vi "GetDiscoveredDevices.vi"(0 "CmdLib In":refnum<k24>, 7 "Master Count":i32, 9 "DeviceKey List":string[](array[string]), 11 "error in":errorcluster) -> (4 "CmdLib Out":refnum<k24>, 6 "Device Array":T1(array[cluster]), 15 "error out":errorcluster)   [LabVIEW 2013]
uses:
  C:/GEECS/Developers Version/source/Device Driver/Picomotor8742dotNet/NewFocus/CmdLib.dll
  CmdLib.dll
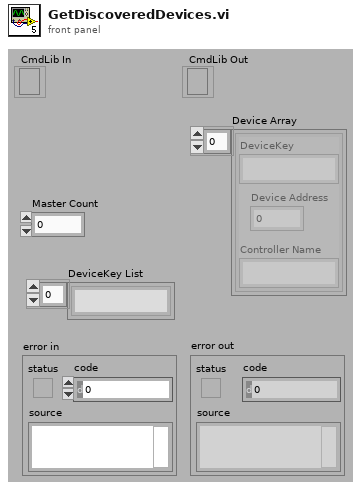
[diagram p1: front panel]
types:
  T1 = cluster{"DeviceKey":string, "Device Address":i32, "Controller Name":string}[]
  T2 = cluster{"DeviceKey Out":string, "Device Address Out":i32, "Controller Name":string}
  T3 = cluster{"DeviceKey Out":string, "Device Address Out":i32, "Controller Name":string}[]
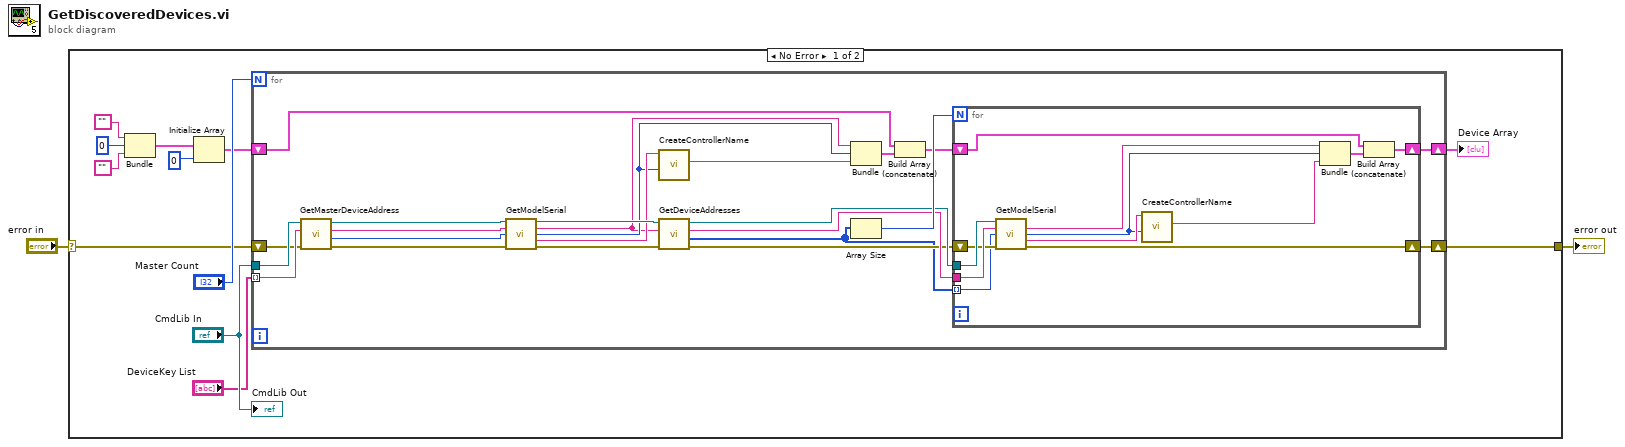
[diagram p0: block diagram]
diagram:
  n1 = case shown="No Error" "error in" {
    selector: "error in" -> [w10 w50]
    tunnel: [w11 w50] -> w2
    frame No Error {
      n2 = Bundle("", 0, "") -> (w6:cluster{string, i32, string})  [unwired: 1 in]
      n3 = Initialize Array(w6, 0 ("dimension size")) -> (w4:cluster{string, i32, string}[])
      n4 = for {
        N: "Master Count" -> [_]
        tunnel: "CmdLib In" -> [w27]
        tunnel: "DeviceKey List" -> [w26] mode=indexing
        shift-right: [w24] -> w11
        shift-left: w10 -> [w25]
        shift-right: [w15] -> w3
        shift-left: w4 -> [w18]
        n5 = call "GetMasterDeviceAddress.vi"("error in (no error)"=w25, "DeviceKey In"=w26, "CmdLib In"=w27) -> ("error out"=w36:errorcluster, "Device Address"=w22:i32, "DeviceKey Out"=w20:string, "CmdLib Out"=w37:refnum<k24>)  [unwired: 1 in]
        n6 = call "GetModelSerial.vi"("CmdLib In"=w37, "DeviceKey In"=w20, "Device Address In"=w22, "error in (no error)"=w36) -> ("CmdLib Out"=w34:refnum<k24>, "DeviceKey Out"=w19:string, "Device Address Out"=w21:i32, "Model / Serial"=w32:string, "error out"=w35:errorcluster)  [unwired: 7 in]
        n7 = call "CreateControllerName.vi"("Device Address"=w21, "Model / Serial"=w32) -> ("Controller Name"=w23:string)  [unwired: 9 in]
        n8 = call "GetDeviceAddresses.vi"("error in (no error)"=w35, "DeviceKey In"=w19, "CmdLib In"=w34) -> ("error out"=w29:errorcluster, "Device Addresses"=w28:i32[], "DeviceKey Out"=w31:string, "CmdLib Out"=w30:refnum<k24>)  [unwired: 1 in]
        n9 = Bundle("DeviceKey Out"=w19, "Device Address Out"=w21, "Controller Name"=w23) -> (w17:T2)  [unwired: 1 in]
        n10 = Array Size(array=w28) -> (size(s)=w33:i32)
        n11 = Build Array (concatenate)(w18, w17) -> (w16:T3)
        n12 = for {
          N: w33 -> [_]
          tunnel: w31 -> [w49]
          tunnel: w30 -> [w48]
          tunnel: w28 -> [w44] mode=indexing
          shift-right: [w47] -> w24
          shift-left: w29 -> [w45]
          shift-right: [w42] -> w15
          shift-left: w16 -> [w43]
          n13 = call "GetModelSerial.vi"("CmdLib In"=w48, "DeviceKey In"=w49, "Device Address In"=w44, "error in (no error)"=w45) -> ("DeviceKey Out"=w38:string, "Device Address Out"=w39:i32, "Model / Serial"=w46:string, "error out"=w47:errorcluster)  [unwired: 7 in, 1 out]
          n14 = call "CreateControllerName.vi"("Device Address"=w39, "Model / Serial"=w46) -> ("Controller Name"=w40:string)  [unwired: 9 in]
          n15 = Bundle("DeviceKey Out"=w38, "Device Address Out"=w39, "Controller Name"=w40) -> (w41:T2)  [unwired: 1 in]
          n16 = Build Array (concatenate)(w43, w41) -> (w42:T3)
        }
      }
      "Device Array" <- w3
      "CmdLib Out" <- "CmdLib In"
    }
    frame Error {
    }
  }
  "error out" <- w2
